vi "Ex-04 Acq Finite Multipoint FFT & Noise Gen.vi"() -> ()   [LabVIEW 2012]
doc: "© Copyright M. Ferrari 2012\nMultipoint Analog Acq. Mean, FFT & Noise Gen"
uses:
  <vilib>/DAQmx/create/channels.llb/DAQmx Create Channel (AI-Voltage-Basic).vi
  <vilib>/DAQmx/configure/timing.llb/DAQmx Timing (Sample Clock).vi
  <vilib>/DAQmx/read.llb/DAQmx Read (Analog Wfm 1Chan NSamp).vi
  <vilib>/express/express analysis/Spectral/XNode/ExpressSpectralMeasurementsBlockNode.xnode
  <vilib>/express/express analysis/Spectral/Block/exnSpectralBlock spectral measurements RMS poly.vi
  <vilib>/express/express analysis/Spectral/Block/exnSpectralBlock spectral measurements RMS WFM.vi
  <vilib>/measure/NI_MABase.lvlib
panel:
  in  "ampiezza rumore":dbl(knob) scale=0.0..5.0
  in  "n° samples":i32=1000
  in  "rate":dbl=10000.0
  in  "min":dbl=-5.0 format="%0.2f"
  in  "max":dbl=5.0 format="%0.2f"
  in  "in conf":i32(ring)=10083 items=["default"=-1, "RSE"=10083, "NRSE"=10078, "Differential"=10106, "Pseudodifferential"=12529]
  in  "physical ch":tag="Dev1/ai0"
  out "FFT":cluster{"f0":dbl, "df":dbl, "magnitude":dbl[]}(graph)
  out "FFT - (RMS)":cluster{"f0":dbl, "df":dbl, "magnitude":dbl[]}
  out "Volt Graph":waveform(dbl)(graph)
  out "MEDIA":dbl format="%0.2f"
  # "RANGE"
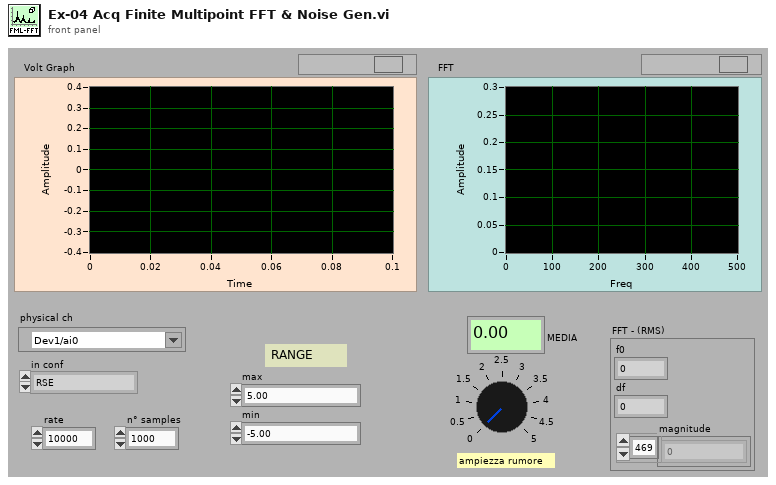
[diagram p1: front panel]
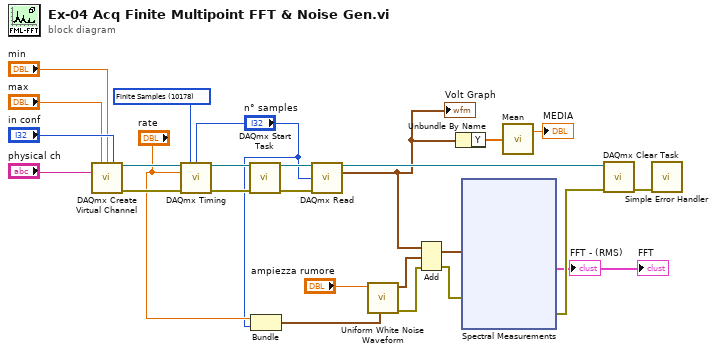
[diagram p0: block diagram]
diagram:
  w19 = 10178 items=["Finite Samples"=10178, "Continuous Samples"=10123, "Hardware Timed Single Point"=12522] ("sample mode")
  n1 = call-poly <vilib>:"DAQmx Create Virtual Channel.vi"("maximum value"="max", "minimum value"="min", "input terminal configuration"="in conf", "physical channels"="physical ch") -> ("task out"=w25:refnum<k21>, "error out"=w24:errorcluster)  [unwired: 5 in, 5 out]
  n2 = call-poly <vilib>:"DAQmx Timing.vi"("task/channels in"=w25, "sample mode"=w19, "samples per channel"="n° samples", "rate"="rate") -> ("task out"=w20:refnum<k21>)  [unwired: 3 in, 8 out]
  n3 = call <vilib>:"DAQmx Start Task.vi"("task/channels in"=w20, "error in"=w24) -> ("task out"=w23:refnum<k21>, "error out"=w22:errorcluster)  [unwired: 12 out]
  n4 = Bundle("rate"="rate", "n° samples"="n° samples") -> (w5:cluster{"rate":dbl, "n° samples":i32})  [unwired: 1 in]
  n5 = call-poly <vilib>:"DAQmx Read.vi"("task/channels in"=w23, "number of samples per channel"="n° samples", "error in"=w22) -> ("task out"=w21:refnum<k21>, "data"=w7:waveform(dbl))  [unwired: 11 out]
  "Volt Graph" <- w7
  n6 = call <vilib>:"Uniform White Noise Waveform.vi"("sampling info"=w5, "amplitude"="ampiezza rumore") -> ("error out"=w2:errorcluster, "signal out"=w8:waveform(dbl))  [unwired: 3 in, 5 out]
  n7 = Add(1:w8, 2:w7, 4:w2) -> (0:w6:waveform(dbl), 3:w1:errorcluster)
  n8 = Unbundle By Name(w7) -> ("Y"=w16:dbl[])
  n9 = xnode "Spectral Measurements"("Signals"=w6, "error in (no error)"=w1) -> ("FFT - (RMS)"=→"FFT - (RMS)" →"FFT":cluster{"f0":dbl, "df":dbl, "magnitude":dbl[]}, "error out"=w15:errorcluster)  [unwired: 1 out]
  n10 = call <vilib>:"Mean.vi"("X"=w16) -> ("mean"=→"MEDIA":dbl)  [unwired: 1 out]
  n11 = call <vilib>:"DAQmx Clear Task.vi"("task in"=w21, "error in"=w15) -> ("error out"=w18:errorcluster)  [unwired: 13 out]
  n12 = call <vilib>:"Simple Error Handler.vi"("error in (no error)"=w18) -> ()  [unwired: 1 in, 8 out]
